vi "MDrive_Init_Com.vi"(8 "error in (no error)":errorcluster, 10 "baud rate":u32=9600, 11 "VISA resource name":refnum<visa-resource-name>="COM6") -> (0 "error out":errorcluster, 3 "VISA resource name out":refnum<visa-resource-name>="COM6")   [LabVIEW 2015]
uses:
  <vilib>/Instr/_visa.llb/VISA Set IO Buffer Mask.ctl
  <vilib>/Instr/_visa.llb/VISA Configure Serial Port (Instr).vi
panel:
  in  "Serial Settings:Wire Mode":i16(ring) items=["Unknown"=-1, "RS485/Wire4"=0, "RS485/Wire2-EchoDTR"=1, "RS485/Wire2-CtrlDTR"=2, "RS485/Wire2-Auto"=3, "RS232/DTE"=128, "RS232/DCE"=129, "RS232/AUTO"=130]
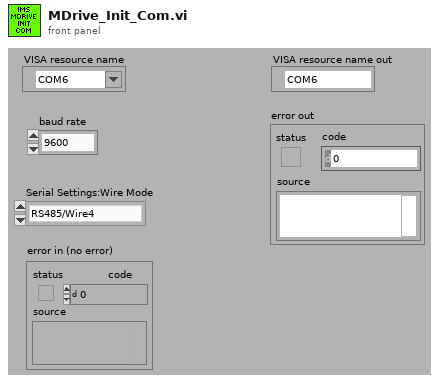
[diagram p1: front panel]
types:
  T1 = typedef "VISA Set IO Buffer Mask.ctl" = u16
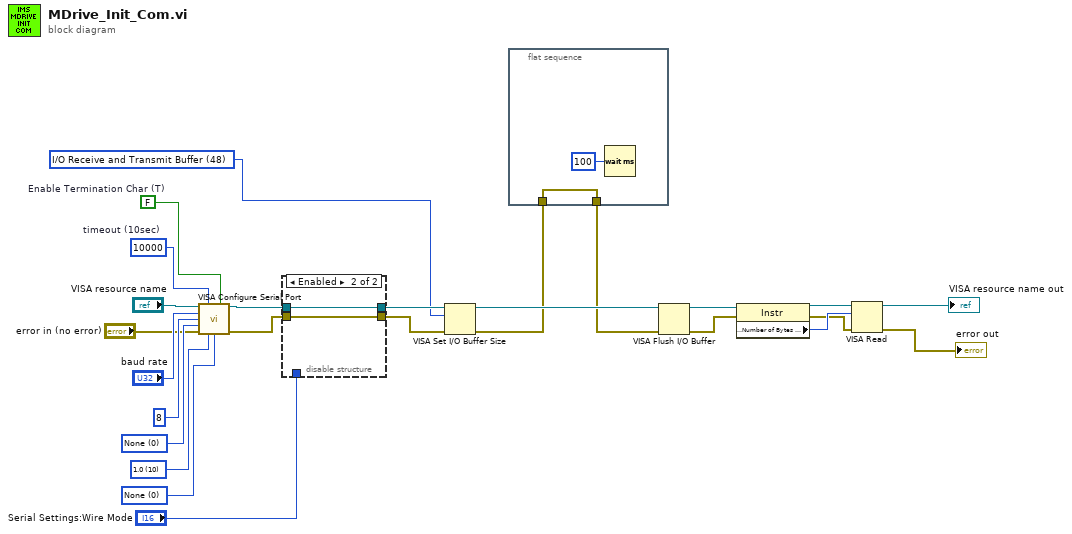
[diagram p0: block diagram]
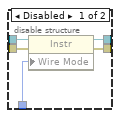
[diagram p2: hidden frame]
diagram:
  w18 = u16 10 items=["1.0"=10, "1.5"=15, "2.0"=20] ("stop bits (10: 1 bit)")
  w20 = u16 0 items=["None", "Odd", "Even", "Mark", "Space"] ("parity")
  w19 = u16 0 items=["None"=0, "XON/XOFF"=1, "RTS/CTS"=2, "DTR/DSR"=4] ("flow control")
  w11 = T1 48 items=["I/O Receive Buffer"=16, "I/O Transmit Buffer"=32, "I/O Receive and Transmit Buffer"=48] ("Mask")
  w25 = FALSE  # Enable Termination Char (T)
  w22 = u32 10000  # timeout (10sec)
  n1 = call-poly "VISA Configure Serial Port"("VISA resource name"="VISA resource name", "timeout (10sec)"=w22, "Enable Termination\nChar (T)"=w25, "baud rate (9600)"="baud rate", "data bits (8)"=u16 8 ("data bits"), "parity (0:none)"=w20, "error in (no error)"="error in (no error)", "stop bits (10: 1 bit)"=w18, "flow control (0:none)"=w19) -> ("VISA resource name out"=w15:refnum<visa-resource-name>, "error out"=w13:errorcluster)  [unwired: 5 out]
  n2 = disable-structure shown="Enabled" {
    disable-tunnel: "Serial Settings:Wire Mode" -> [w30 _]
    disable-tunnel: w15 -> [w29 w32]
    disable-tunnel: [w28 w32] -> w14
    disable-tunnel: w13 -> [w27 w31]
    disable-tunnel: [w26 w31] -> w12
    frame Disabled {
      n3 = property class="Instr"(reference=w29, error in=w27, "Wire Mode"=w30) -> (reference out=w28:refnum<visa-resource-name>, error out=w26:errorcluster)
    }
    frame Enabled {
    }
  }
  n4 = VISA Set I/O Buffer Size(VISA resource name=w14, mask (16)=w11, error in (no error)=w12) -> (VISA resource name out=w16:refnum<visa-resource-name>, error out=w9:errorcluster)  [unwired: 1 in]
  n5 = flat-sequence {
    tunnel: w9 -> [w33]
    tunnel: [w33] -> w8
    frame #0 {
      n6 = Wait (ms)(milliseconds to wait=u32 100) -> ()  [unwired: 1 out]
    }
  }
  n7 = VISA Flush I/O Buffer(VISA resource name=w16, error in (no error)=w8) -> (VISA resource name out=w10:refnum<visa-resource-name>, error out=w7:errorcluster)  [unwired: 1 in]
  n8 = property class="Instr"(reference=w10, error in=w7) -> (reference out=w6:refnum<visa-resource-name>, error out=w4:errorcluster, "Serial Settings:Number of Bytes at Serial Port"=w5:u32)
  n9 = VISA Read(VISA resource name=w6, byte count=w5, error in (no error)=w4) -> (VISA resource name out=→"VISA resource name out":refnum<visa-resource-name>, error out=→"error out":errorcluster)  [unwired: 2 out]
